vi "多列列表框-插入项名.vi"(8 "插入位置（T首，F尾）":bool=TRUE, 9 "项名(整行)":string[](array[string]), 10 "限定行数":u32, 11 "MCListbox引用句柄":refnum<vi>) -> (3 "引用输出":refnum<vi>)   [LabVIEW 2017]
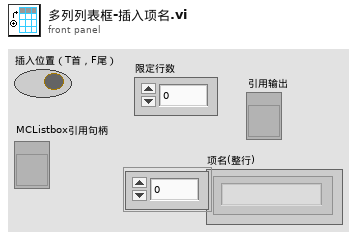
[diagram p1: front panel]
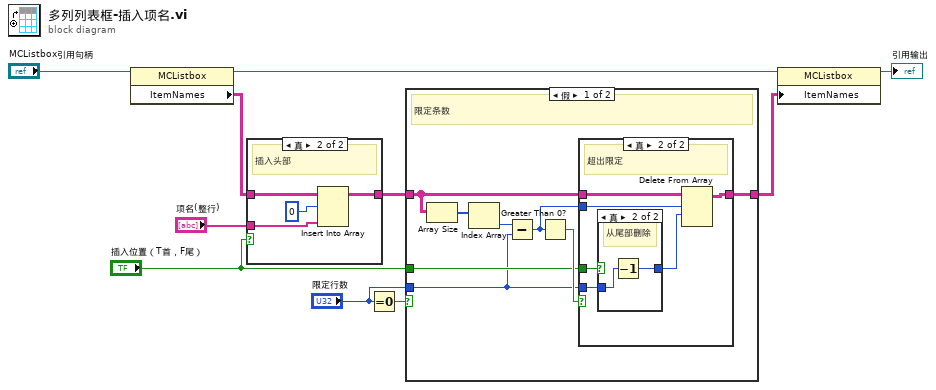
[diagram p0: block diagram]
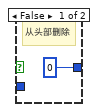
[diagram p3: hidden frame]
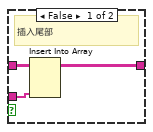
[diagram p5: hidden frame]
diagram:
  n1 = property class="MCListbox"(reference="MCListbox引用句柄") -> (reference out=w9:refnum<vi>, "ItemNames"=w7:string[][])  [unwired: 1 in, 1 out]
  n2 = case shown="真" "插入位置（T首，F尾）" {
    tunnel: [w13 w15] -> w5
    tunnel: w7 -> [w12 w16]
    tunnel: "项名(整行)" -> [w11 w14]
    frame False {
      # "插入尾部"
      n3 = Insert Into Array(array=w12, new element=w11) -> (w13:string[][])  [unwired: 2 in]
    }
    frame True {
      # "插入头部"
      n4 = Insert Into Array(array=w16, index (row)=0 ("索引"), new element=w14) -> (w15:string[][])  [unwired: 1 in]
    }
  }
  n5 = Equal To 0?(x="限定行数") -> (x = 0?=w2:bool)
  n6 = case shown="假" w2 {
    tunnel: w5 -> [w21 w36]
    tunnel: "限定行数" -> [w22 _]
    tunnel: "插入位置（T首，F尾）" -> [w24 _]
    tunnel: [w20 w36] -> w4
    frame False {
      # "限定条数"
      n7 = Array Size(array=w21) -> (size(s)=w19:i32[])
      n8 = Index Array(array=w19) -> (element=w18:i32)  [unwired: 1 in]
      n9 = Subtract(x=w18, y=w22) -> (x-y=w23:u32)
      n10 = Greater Than 0?(x=w23) -> (x > 0?=w25:bool)
      n11 = case shown="真" w25 {
        tunnel: w24 -> [_ w32]
        tunnel: w23 -> [_ w30]
        tunnel: w22 -> [_ w29]
        tunnel: w21 -> [w26 w28]
        tunnel: [w26 w27] -> w20
        frame False {
          # "未超出"
        }
        frame True {
          # "超出限定"
          n12 = case shown="真" w32 {
            tunnel: [0 ("索引") w34] -> w31
            tunnel: w29 -> [_ w35]
            frame False {
              # "从头部删除"
            }
            frame True {
              # "从尾部删除"
              n13 = Decrement(x=w35) -> (x-1=w34:u32)
            }
          }
          n14 = Delete From Array(array=w28, length=w30, index (row)=w31) -> (array with subset deleted=w27:string[][])  [unwired: 1 in, 1 out]
        }
      }
    }
    frame True {
      # "未限定条数"
    }
  }
  n15 = property class="MCListbox"(reference=w9, "ItemNames"=w4) -> (reference out=→"引用输出":refnum<vi>)  [unwired: 1 in, 1 out]
